vi "LinearFilter_MovingAverage.vi"(11 "Samples":i32=1 min=1) -> (3 "LINEAR_FILTER":T1 {"Outputs" format="%13.5p"; "Inputs" format="%13.5p"; "OutputGains" format="%13.5p"; "InputGains" format="%13.5p"})   [LabVIEW 2019, in "Trajectory_Library.lvlib"]
doc: "Creates a K-tap FIR moving average filter of the form: \n\n y[n] = 1/k * (x[k] + x[k-1] + ... + x[0]).\n \nThis filter is always stable.\n \nInputs: \n - Samples - The number of samples to average over. Higher = smoother but slower.\n The number of samples must be >= 1\n\nOutputs:\n - Linearfilter - Created datat structure"
uses:
  Trajectory_Library.lvlib
  LINEAR_FILTER.ctl
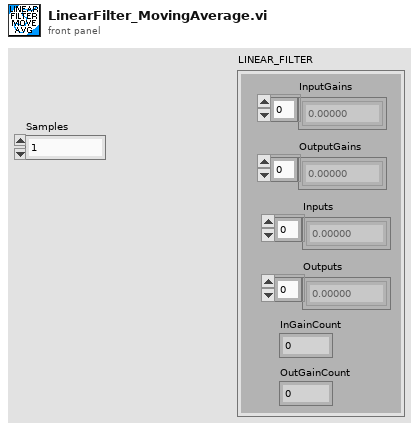
[diagram p1: front panel]
types:
  T1 = typedef "Trajectory_Library.lvlib/LINEAR_FILTER.ctl" = cluster{"InputGains":dbl[], "OutputGains":dbl[], "Inputs":dbl[], "Outputs":dbl[], "InGainCount":i32, "OutGainCount":i32}
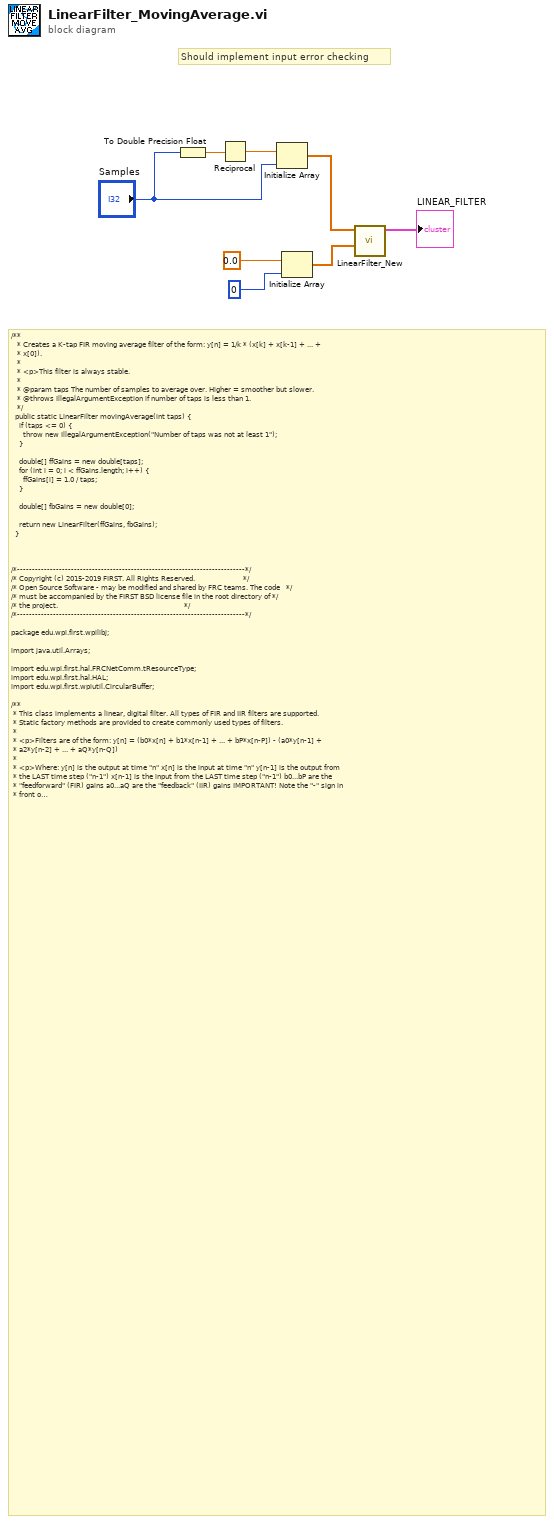
[diagram p0: block diagram]
diagram:
  # "Should implement input error checking"
  # "/**\n   * Creates a K-tap FIR moving average filter of the form: y[n] = 1/k * (x[k] + x[k-1] + ... +\n   * x[0]).\n   *\n   * <p>This filter is always stable.\n   *\n   * @param taps The number of samples to average over. Higher = smoother but slower.\n   * @throws IllegalArgumentException if number of taps is less than 1.\n   */\n  public static LinearFilter movingAverage(int taps) {\n    if (taps <= 0) {\n      throw new IllegalArgumentException(\"Number of taps was not at least 1\");\n    }\n\n    double[] ffGains = new double[taps];\n    for (int i = 0; i < ffGains.length; i++) {\n      ffGains[i] = 1.0 / taps;\n    }\n\n    double[] fbGains = new double[0];\n\n    return new LinearFilter(ffGains, fbGains);\n  }\n\n\n\n/*----------------------------------------------------------------------------*/\n/* Copyright (c) 2015-2019 FIRST. All Rights Reserved.                        */\n/* Open Source Software - may be modified and shared by FRC teams. The code   */\n/* must be accompanied by the FIRST BSD license file in the root directory of */\n/* the project.                                                               */\n/*----------------------------------------------------------------------------*/\n\npackage edu.wpi.first.wpilibj;\n\nimport java.util.Arrays;\n\nimport edu.wpi.first.hal.FRCNetComm.tResourceType;\nimport edu.wpi.first.hal.HAL;\nimport edu.wpi.first.wpiutil.CircularBuffer;\n\n/**\n * This class implements a linear, digital filter. All types of FIR and IIR filters are supported.\n * Static factory methods are provided to create commonly used types of filters.\n *\n * <p>Filters are of the form: y[n] = (b0*x[n] + b1*x[n-1] + ... + bP*x[n-P]) - (a0*y[n-1] +\n * a2*y[n-2] + ... + aQ*y[n-Q])\n *\n * <p>Where: y[n] is the output at time \"n\" x[n] is the input at time \"n\" y[n-1] is the output from\n * the LAST time step (\"n-1\") x[n-1] is the input from the LAST time step (\"n-1\") b0...bP are the\n * \"feedforward\" (FIR) gains a0...aQ are the \"feedback\" (IIR) gains IMPORTANT! Note the \"-\" sign in\n * front of the feedback term! This is a common convention in signal processing.\n *\n * <p>What can linear filters do? Basically, they can filter, or diminish, the effects of\n * undesirable input frequencies. High frequencies, or rapid changes, can be indicative of sensor\n * noise or be otherwise undesirable. A \"low pass\" filter smooths out the signal, reducing the\n * impact of these high frequency components.  Likewise, a \"high pass\" filter gets rid of\n * slow-moving signal components, letting you detect large changes more easily.\n *\n * <p>Example FRC applications of filters: - Getting rid of noise from an analog sensor input (note:\n * the roboRIO's FPGA can do this faster in hardware) - Smoothing out joystick input to prevent the\n * wheels from slipping or the robot from tipping - Smoothing motor commands so that unnecessary\n * strain isn't put on electrical or mechanical components - If you use clever gains, you can make a\n * PID controller out of this class!\n *\n * <p>For more on filters, we highly recommend the following articles:<br>\n * https://en.wikipedia.org/wiki/Linear_filter<br>\n * https://en.wikipedia.org/wiki/Iir_filter<br>\n * https://en.wikipedia.org/wiki/Fir_filter<br>\n *\n * <p>Note 1: calculate() should be called by the user on a known, regular period. You can use a\n * Notifier for this or do it \"inline\" with code in a periodic function.\n *\n * <p>Note 2: For ALL filters, gains are necessarily a function of frequency. If you make a filter\n * that works well for you at, say, 100Hz, you will most definitely need to adjust the gains if you\n * then want to run it at 200Hz! Combining this with Note 1 - the impetus is on YOU as a developer\n * to make sure calculate() gets called at the desired, constant frequency!\n */"
  n1 = To Double Precision Float(number="Samples") -> (double precision float=w6:dbl)
  n2 = Reciprocal(x=w6) -> (1/x=w5:dbl)
  n3 = Initialize Array(w5, "Samples") -> (w2:dbl[])
  n4 = Initialize Array(0.0, 0) -> (w1:dbl[])
  n5 = call "LinearFilter_New.vi"("OutputGains"=w1, "InputGains"=w2) -> ("LINEAR_FILTER"=→"LINEAR_FILTER":T1)  [unwired: 9 in]
